vi "main.vi"() -> ()   [LabVIEW 2019]
panel:
  in  "Side Menu":enum32{"Page 1", "Page 2"}(tab)
  in  "Slide Menu":enum32{"Page 1", "Page 2"}(tab)
  in  "PosProcessamento":bool
  in  "Calibracao":bool
  in  "Grafico":bool
  in  "[ESC]":bool
  in  "Main tab":T1(tab)
  out "C Graph 2":dbl[](graph)
  out "C Graph":dbl[][](graph)
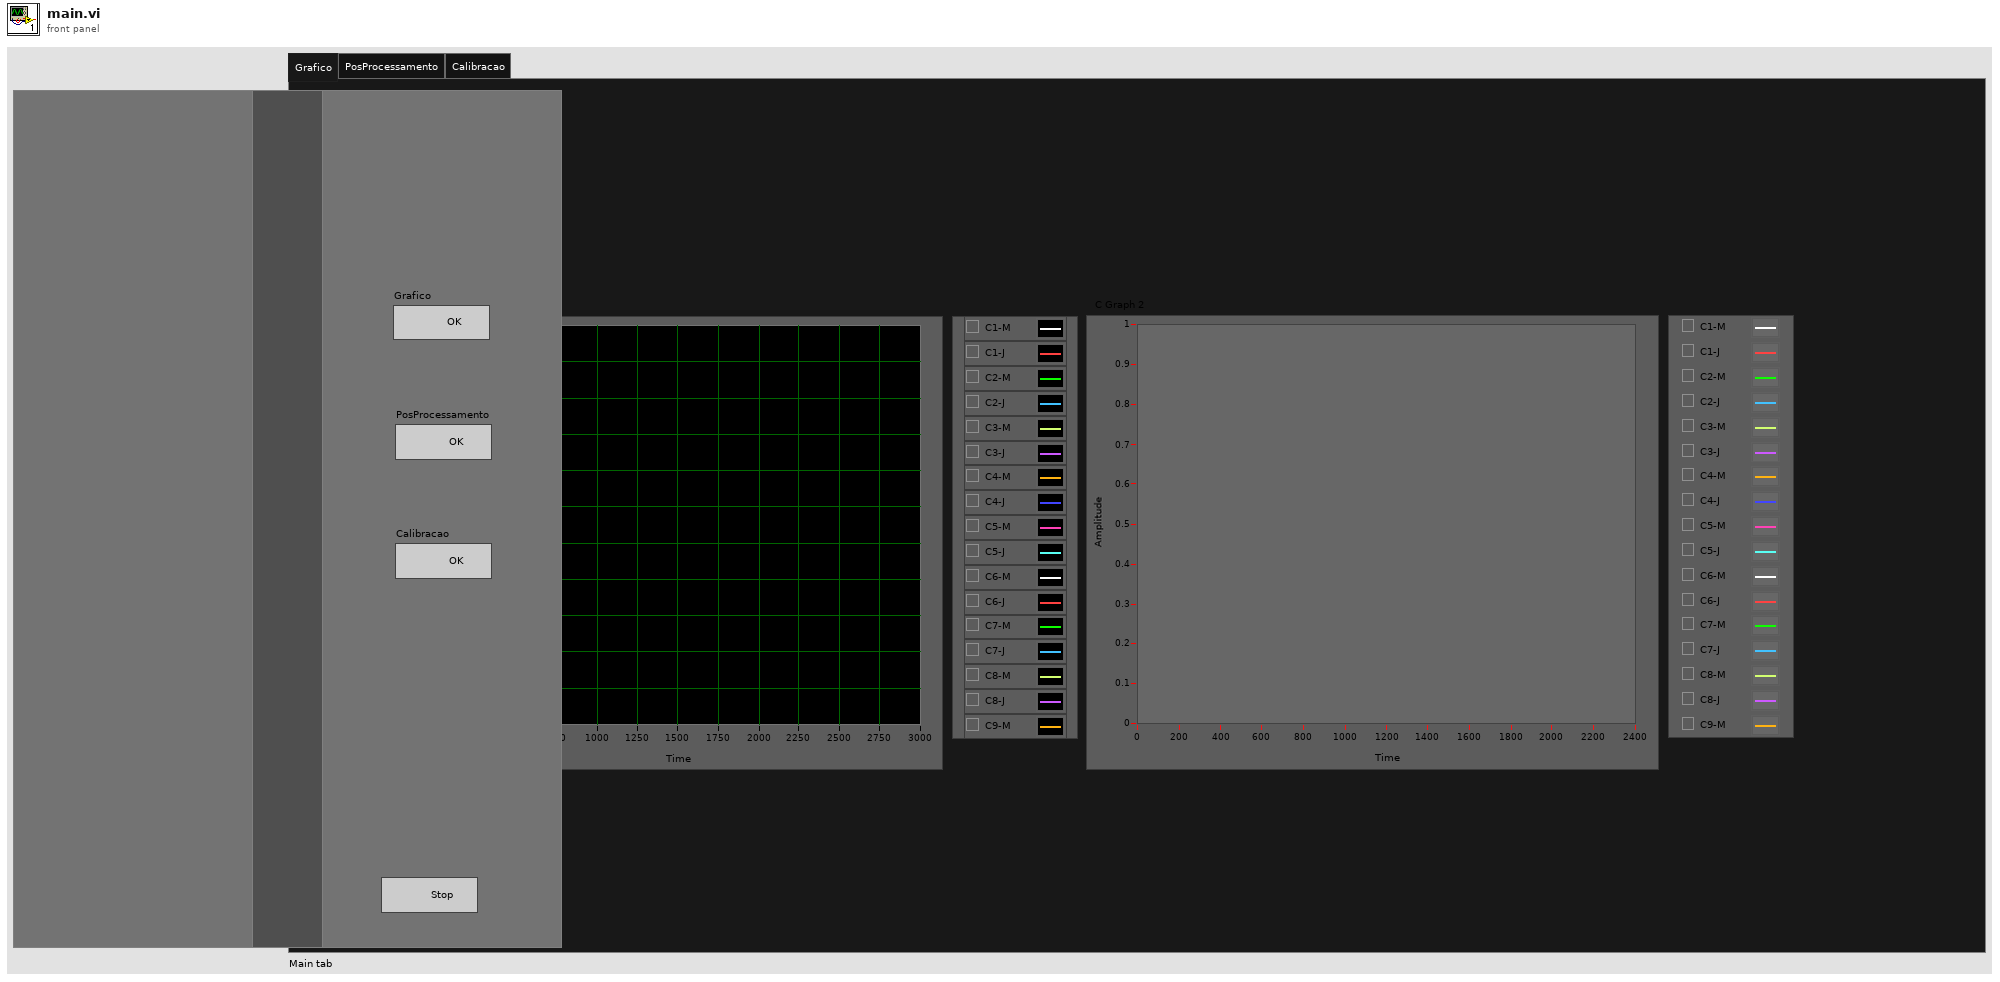
[diagram p1: front panel]
types:
  T1 = enum32{"Grafico", "PosProcessamento", "Calibracao"}
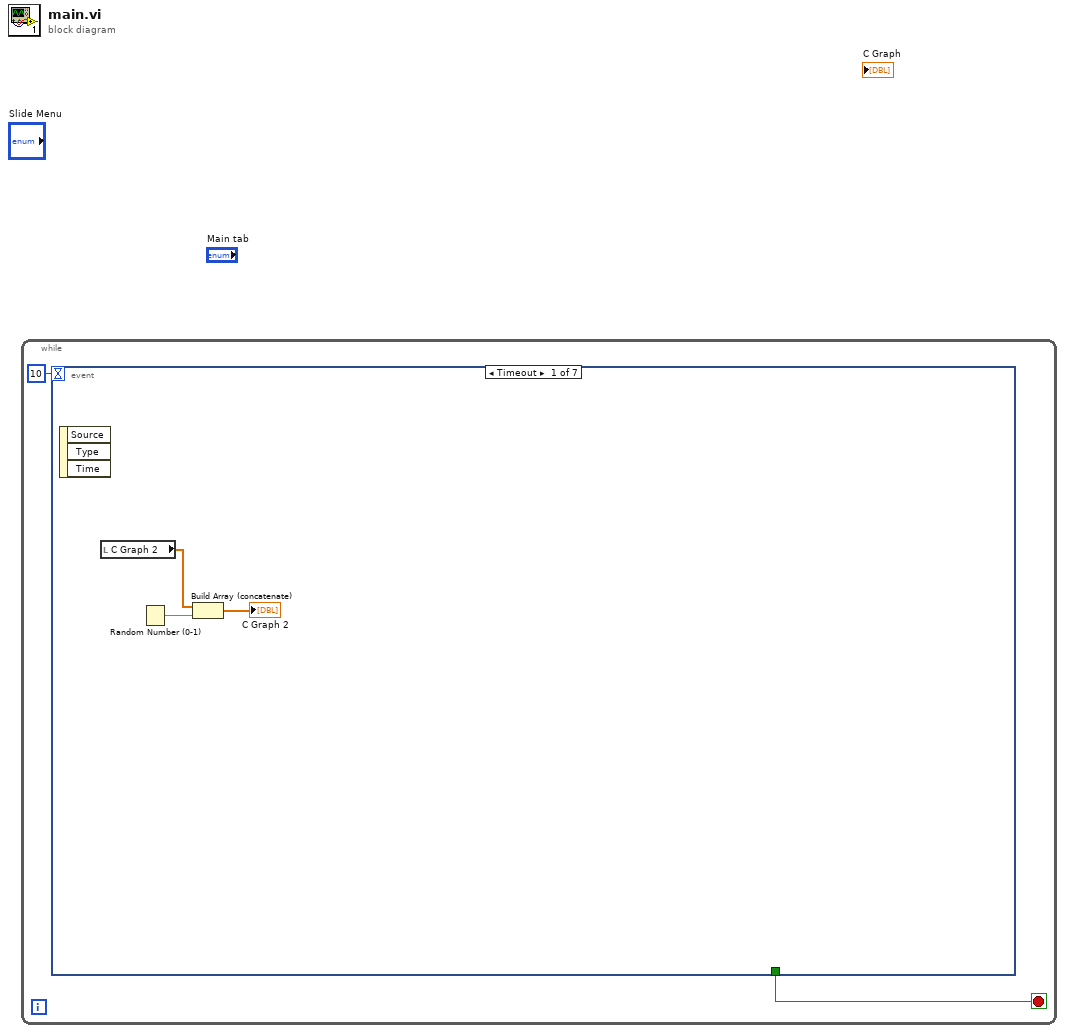
[diagram p0: block diagram]
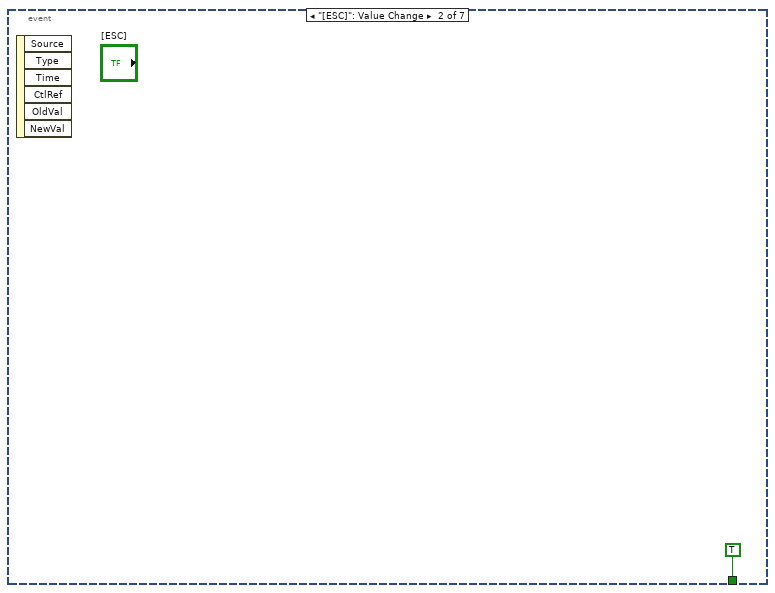
[diagram p2: hidden frame]
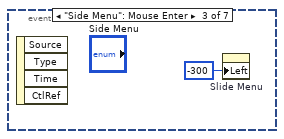
[diagram p3: hidden frame]
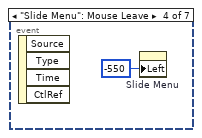
[diagram p4: hidden frame]
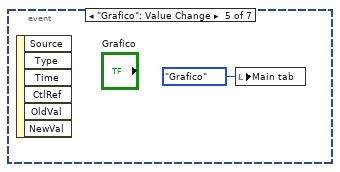
[diagram p5: hidden frame]
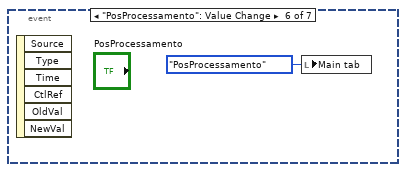
[diagram p6: hidden frame]
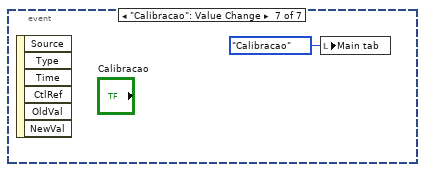
[diagram p7: hidden frame]
diagram:
  n1 = while {
    stop <- w2 stop-if-true
    n2 = event shown="[0] Timeout" {
      selector: _ -> [_ _ _ _ _ _ _]
      dyn-events: _ -> [_ _ _ _ _ _ _]
      timeout: 10 -> [_ _ _ _ _ _ _]
      tunnel: [_ TRUE ("Stop Button") _ _ _ _ _] -> w2
      event Timeout {
        n3 = event-data() -> ()  [unwired: 1 in, 3 out]
        n4 = local read "C Graph 2"() -> (w3:dbl[])
        n5 = Random Number (0-1)() -> (number: 0 to 1=w5:dbl)
        n6 = Build Array (concatenate)(w3, w5) -> (→"C Graph 2":dbl[])
      }
      event "[ESC]": Value Change {
        n7 = event-data() -> ()  [unwired: 1 in, 6 out]
      }
      event "Side Menu": Mouse Enter {
        n8 = event-data() -> ()  [unwired: 1 in, 4 out]
        n9 = property on="Slide Menu" class="TabCtl (strict)"("Left"=-300 ("Position:Left")) -> ()  [unwired: 2 in, 2 out]
      }
      event "Slide Menu": Mouse Leave {
        n10 = event-data() -> ()  [unwired: 1 in, 4 out]
        n11 = property on="Slide Menu" class="TabCtl (strict)"("Left"=-550 ("Position:Left")) -> ()  [unwired: 2 in, 2 out]
      }
      event "Grafico": Value Change {
        n12 = event-data() -> ()  [unwired: 1 in, 6 out]
        n13 = local write "Main tab"(T1."Grafico" ("Main tab")) -> ()
      }
      event "PosProcessamento": Value Change {
        n14 = event-data() -> ()  [unwired: 1 in, 6 out]
        n15 = local write "Main tab"(T1."PosProcessamento" ("Main tab")) -> ()
      }
      event "Calibracao": Value Change {
        n16 = event-data() -> ()  [unwired: 1 in, 6 out]
        n17 = local write "Main tab"(T1."Calibracao" ("Main tab")) -> ()
      }
    }
  }
